vi "Ixon z-stack acquisition.vi"() -> ()   [LabVIEW 2015]
doc: "Acquires a z-stack of images using the Andor iXon camera and the piezo stage. The VI can be configured to sequentially acquire frames in multiple modes with different light sources and numbers of frames in each mode. Each mode is collected into a separate aquisition directory in Glimpse. Acquisition can be time-lapsed with a settable delay interval between cycles; the selected laser(s) are shuttered whilst not acquiring. The ixon setup acquisition.vi front panel is displayed so that the user can set the acquisition parameters before acquiring.\n\nThis is a Glimpse plug-in. To insure proper operation, you should have the source version of Glimpse running before loading this program. (The source version has an .llb extension, not a .exe one). Alternatively, the plug-in can be inserted into the executable version of Glimpse as a dynamically loaded VI."
uses:
  Glimpse core/Video acquisition state.ctl
  <vilib>/vision/Image Controls.llb/IMAQ Image.ctl
  Glimpse core/Seq file v 1/Offset table.ctl
  Glimpse core/Seq file v 1/file number.ctl
  Glimpse core/Seq file v 1/Offset.ctl
  Glimpse core/GLIMPSE Globals.vi
  ixon1024/camera defaults globals.vi
  Camera/camera globals.vi
  Stage/Move stage command.ctl
  ixon1024/ixon readout settings.ctl
  ixon1024/andor acquisition mode.ctl
  ixon1024/HAL camera parameters important.ctt
  new-h-nu-ixon/Laser type.ctt
  new-h-nu-ixon/Emission filters.ctl
panel:
  in  "Delay after\nfilter change\n(ms)":u32
  in  "Max. number of acquisition files":i8(slide)=10 scale=0.0..50.0
  in  "Camera Parameters":T1={"Exposure Time (sec)"=0.1, "EM CCD Gain"=230, "Readout Settings"={"Acquisition Mode"=enum."Frame Transfer Run till Abort", "Pixel Rate"=enum."EM CCD 5 Mhz 14 bits", "High Capacity?"=FALSE, "V Shift Speed (us/row)"=enum."6.5", "V Shift Amplitude"=enum."+1", "Preamp Gain"=enum."2.4", "Trigger Mode"=0, "Baseline offset"=0, "Baseline clamp"=FALSE}, "Image Size"={"H Bin"=1, "V Bin"=1, "Left"=1, "Top"=1, "Right"=1024, "Bottom"=730}} {"Readout Settings"."Baseline offset" min=-1000 max=1000 step=100; "Readout Settings"."Trigger Mode" items=["Internal", "External"]; "EM CCD Gain" scale=1.0..300.0; "Exposure Time (sec)" scale=0.001..10.0 scale format="%#_1g"}
  in  "stage settle time (ms)":u32=300
  in  "stack half-width (steps)":u32=8
  in  "focus step (um)":ext=0.150000000000000000005
  in  "Cycle Interval (s)":dbl format="%_3f"
  in  "Acquisition Protocol":T6(array[cluster])
  # "Z-stack parameters"
  # "Camera: Andor iXon"
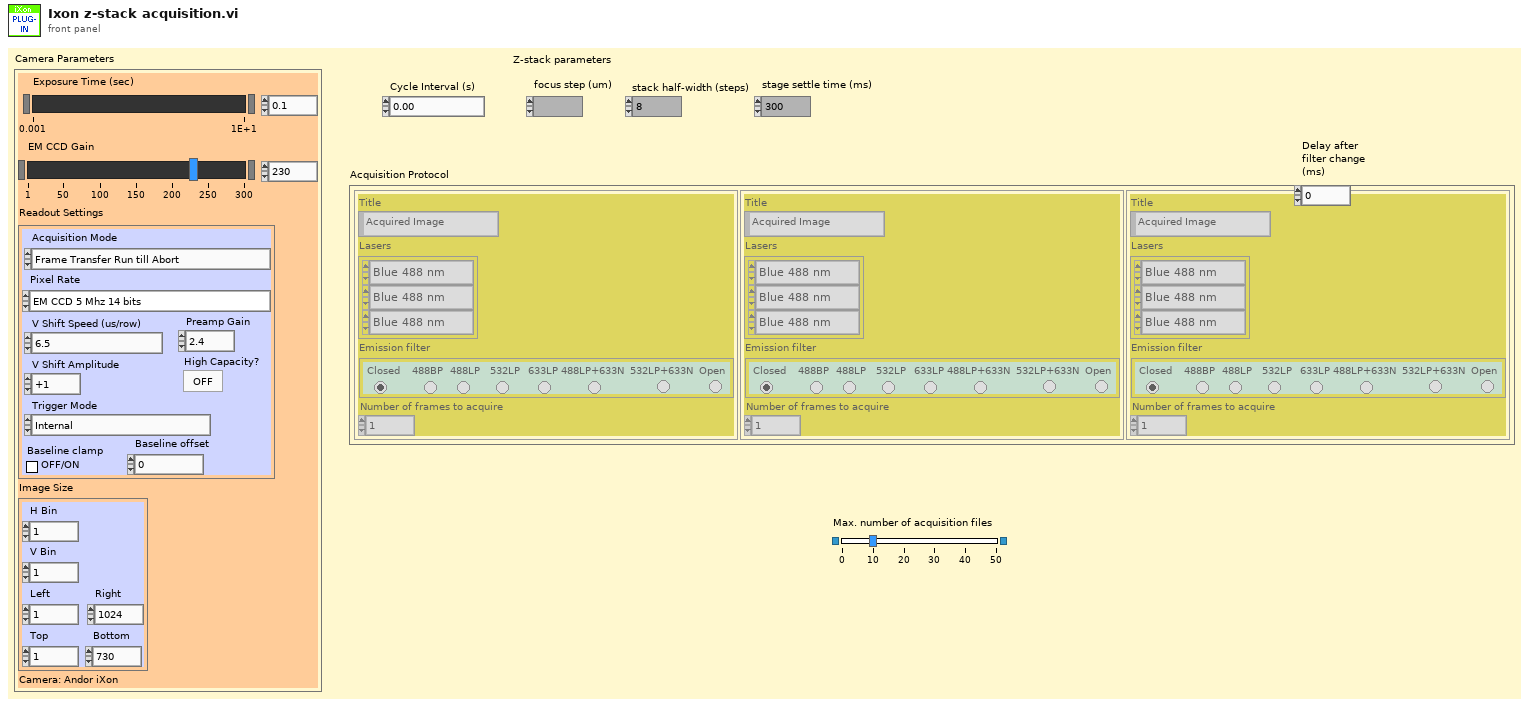
[diagram p1: front panel]
types:
  T1 = typedef "HAL camera parameters important.ctt" = cluster{"Exposure Time (sec)":sgl, "EM CCD Gain":u16, "Readout Settings":T2, "Image Size":cluster{"H Bin":i32, "V Bin":i32, "Left":i32, "Top":i32, "Right":i32, "Bottom":i32}}
  T2 = typedef "ixon readout settings.ctl" = cluster{"Acquisition Mode":T3, "Pixel Rate":enum16{"EM CCD 10 Mhz 14 bits", "EM CCD 5 Mhz 14 bits", "EM CCD 3 Mhz 14 bits", "EM CCD 1 Mhz 16 bits", "Standard CCD 3 Mhz 14 bits", "Standard CCD 1 Mhz 16 bits"}, "High Capacity?":bool, "V Shift Speed (us/row)":enum16{"0.9 (not reccommended)", "1.7  (not reccommended)", "3.3  (not reccommended)", "6.5", "12.9"}, "V Shift Amplitude":enum16{"normal", "+1", "+2", "+3", "+4"}, "Preamp Gain":enum16{"1.0", "2.4", "5.0"}, "Trigger Mode":u32, "Baseline offset":i16, "Baseline clamp":bool}
  T3 = typedef "andor acquisition mode.ctl" = enum16{"(do not use)", "Single Scan", "Accumulate", "Kinetics", "Fast Kinetics", "Kinetics Run till Abort", "Frame Transfer", "Frame Transfer Run till Abort", "(do not use) ", "Time Delayed Integration"}
  T4 = typedef "Laser type.ctt" = enum16{"Blue 488 nm", "Green 532 nm", "Red 633 nm", "IR 780"}
  T5 = typedef "Emission filters.ctl" = enum32{" Closed ", " 488BP ", "488LP", "  532LP ", "633LP", "488LP+633N", "532LP+633N", "Open"}
  T6 = cluster{"Title":string, "Lasers":T4[], "Emission filter":T5, "Number of frames to acquire":i32}[]
  T7 = typedef "image size.ctl" = cluster{"H Bin":i32, "V Bin":i32, "Left":i32, "Top":i32, "Right":i32, "Bottom":i32}
  T8 = typedef "Glimpse file parameters.ctt" = cluster{"Frame Size (bytes)":u32, "Max Frames":u32, "Max time (s)":u32, "Max Time (min)":u32, "Max Space Req'd. (Gb)":dbl, "Frames per acquisition file":u32}
  T9 = typedef "Move stage command.ctl" = cluster{"dx (um) (0 -> ignore)":ext, "dy (um) (0 -> ignore)":ext, "dz (um) (0 -> ignore)":ext, "Re-center x,y":bool, "Re-center z":bool, "x (um) (-1 -> ignore)":dbl, "y (um) (-1 -> ignore)":dbl, "z (um) (-1 -> ignore)":dbl}
  T10 = typedef "Video acquisition state.ctl" = cluster{"Pixel depth":enum32{"8 bits", "16 bits", "Float", "Complex", "RGB Chunky", "Compressed"}, "Width":dbl, "Height":dbl, "Buffer":T11, "Frames Acquired":u32, "Time of 1st frame":dbl, "TTB element zero":u32, "File Offsets Array":T12, "TTB Array":u32[], "Sum Image (for averaging)":T11, "Time at end of last acquisition (ms)":u32, "Filter array":u16[], "Flow rate array":dbl[], "Temperature array":dbl[], "Field array":u16[], "Lasers array":u16[][], "Stage xyz array":dbl[][]}
  T11 = typedef "IMAQ Image.ctl" = refnum<image>
  T12 = typedef "Offset table.ctl" = cluster{"offset":T13, "file number":T14}[]
  T13 = typedef "Offset.ctl" = i32
  T14 = typedef "file number.ctl" = u8
  T15 = typedef "Sequence files handle.ctt" = cluster{"Sequence files directory path":path, "Sequence files refnum array":refnum<file>[]}
  T16 = cluster{"dx (um)":ext, "dy (um)":ext, "dz (um)":ext}
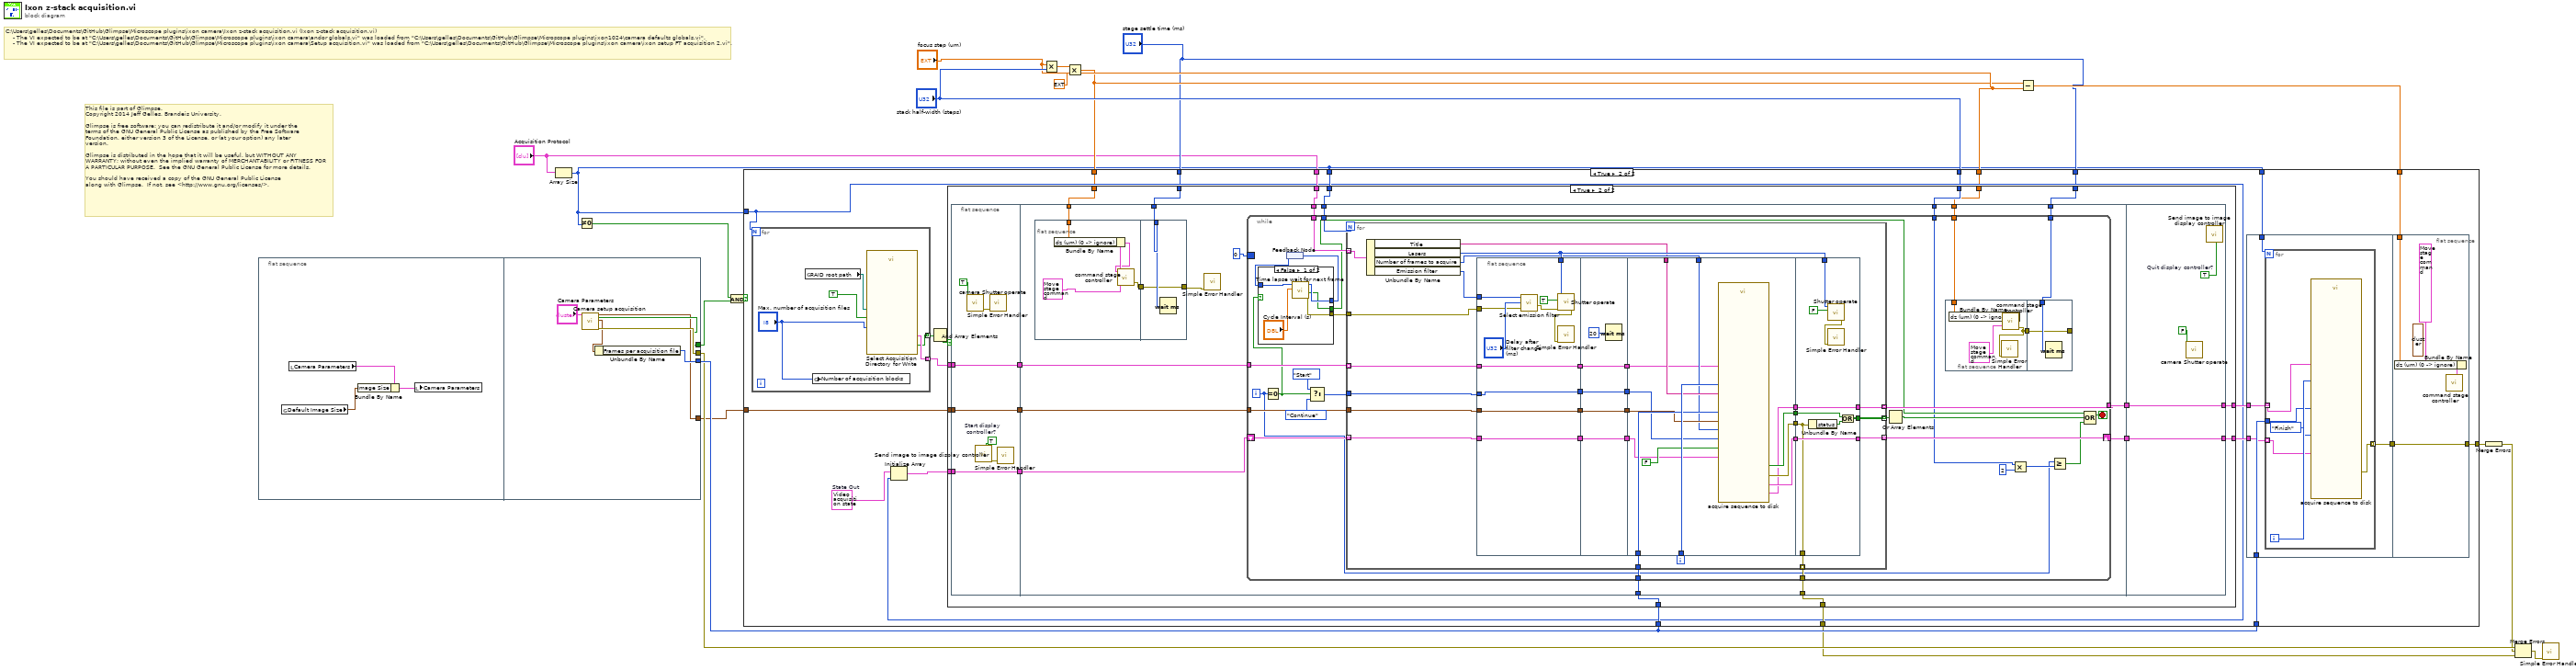
[diagram p0: block diagram]
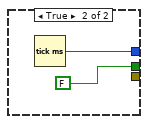
[diagram p4: hidden frame]
diagram:
  # "C:\\Users\\gelles\\Documents\\GitHub\\Glimpse\\Microscope plugins\\ixon camera\\Ixon z-stack acquisition.vi (Ixon z-stack acquisition.vi)\n    - The VI expected to be at \"C:\\Users\\gelles\\Documents\\GitHub\\Glimpse\\Microscope plugins\\ixon camera\\andor globals.vi\" was loaded from \"C:\\Users\\gelles\\Documents\\GitHub\\Glimpse\\Microscope plugins\\ixon1024\\camera defaults globals.vi\".\n    - The VI expected to be at \"C:\\Users\\gelles\\Documents\\GitHub\\Glimpse\\Microscope plugins\\ixon camera\\Setup acquisition.vi\" was loaded from \"C:\\Users\\gelles\\Documents\\GitHub\\Glimpse\\Microscope plugins\\ixon camera\\ixon setup FT acquisition 2.vi\"."
  # "This file is part of Glimpse. \nCopyright 2014 Jeff Gelles, Brandeis University.    \n\nGlimpse is free software: you can redistribute it and/or modify it under the \nterms of the GNU General Public License as published by the Free Software \nFoundation, either version 3 of the License, or (at your option) any later \nversion.\n\nGlimpse is distributed in the hope that it will be useful, but WITHOUT ANY \nWARRANTY; without even the implied warranty of MERCHANTABILITY or FITNESS FOR \nA PARTICULAR PURPOSE.  See the GNU General Public License for more details.\n\nYou should have received a copy of the GNU General Public License\nalong with Glimpse.  If not, see <http://www.gnu.org/licenses/>."
  n1 = flat-sequence {
    tunnel: [w24] -> w11
    tunnel: [w27] -> w10
    tunnel: [w26] -> w4
    tunnel: [w23] -> w1
    frame #0 {
      n2 = global read "camera defaults globals.vi" "Default Image Size"() -> (w22:T7)
      n3 = local read "Camera Parameters"() -> (w21:T1)
      n4 = Bundle By Name(cluster=w21, "Image Size"=w22) -> (w20:T1)
      n5 = local write "Camera Parameters"(w20) -> ()
    }
    frame #1 {
      n6 = call "Camera setup acquisition.vi"("Camera Parameters (important)"="Camera Parameters") -> ("Image Size Out"=w23:T7, "Continue with acq?"=w26:bool, "Glimpse file properties"=w25:T8, "Error Out (no error)"=w27:errorcluster)  [unwired: 6 in, 9 out]
      n7 = Unbundle By Name(w25) -> ("Frames per acquisition file"=w24:u32)
    }
  }
  n8 = Array Size(array="Acquisition Protocol") -> (size(s)=w3:i32)
  n9 = Not Equal To 0?(x=w3) -> (x != 0?=w2:bool)
  n10 = And(x=w2, y=w4) -> (x .and. y?=w5:bool)
  n11 = Multiply(x="focus step (um)", y="stack half-width (steps)") -> (x*y=w19:ext)
  n12 = Multiply(x=w19, y=ext -1.0) -> (x*y=w14:ext)
  n13 = Subtract(x=w14, y="focus step (um)") -> (x-y=w15:ext)
  n14 = case shown="True" w5 {
    tunnel: w11 -> [_ w50]
    tunnel: w11 -> [_ w49]
    tunnel: [_ w48] -> w8
    tunnel: [_ w47] -> w9
    tunnel: w3 -> [_ w37]
    tunnel: w3 -> [_ w43]
    tunnel: w3 -> [_ w40]
    tunnel: "Acquisition Protocol" -> [_ w38]
    tunnel: w1 -> [_ w36]
    tunnel: "stack half-width (steps)" -> [_ w35]
    tunnel: "stage settle time (ms)" -> [_ w34]
    tunnel: "focus step (um)" -> [_ w33]
    tunnel: w15 -> [_ w31]
    tunnel: w14 -> [_ w30]
    tunnel: "stage settle time (ms)" -> [_ w29]
    frame False {
    }
    frame True {
      w42 = T10 {"Pixel depth"=enum."8 bits", "Width"=0.0, "Height"=0.0, "Buffer"=refnum, "Frames Acquired"=0, "Time of 1st frame"=0.0, "TTB element zero"=0, "File Offsets Array"=[], "TTB Array"=[], "Sum Image (for averaging)"=refnum, "Time at end of last acquisition (ms)"=0, "Filter array"=[], "Flow rate array"=[], "Temperature array"=[], "Field array"=[], "Lasers array"=[], "Stage xyz array"=[]}  # State Out
      n15 = for {
        N: w37 -> [_]
        tunnel: [w231] -> w39 mode=indexing
        tunnel: [w230] -> w51 mode=indexing
        n16 = global read "GLIMPSE Globals.vi" "RAID root path"() -> (w233:path)
        n17 = global write "camera globals.vi" "Number of acquisition blocks"("Max. number of acquisition files") -> ()
        n18 = call "Select Acquisition Directory for Write.vi"("Autostart?"=TRUE, "Acquisition directory root path"=w233, "Number of acquisition files"="Max. number of acquisition files") -> ("Sequence files handle"=w231:T15, "OK?"=w230:bool)  [unwired: 11 in]
      }
      n19 = Initialize Array(w42, w37) -> (w41:T10[])
      n20 = And Array Elements(Boolean array=w51) -> (logical AND=w44:bool)
      n21 = case shown="True" w44 {
        tunnel: [w67 w87] -> w46
        tunnel: w39 -> [w67 w86]
        tunnel: w50 -> [_ w85]
        tunnel: [w68 w84] -> w45
        tunnel: [_ w83] -> w48
        tunnel: w43 -> [_ w82]
        tunnel: w41 -> [w68 w81]
        tunnel: w38 -> [_ w80]
        tunnel: w36 -> [_ w75]
        tunnel: w35 -> [_ w73]
        tunnel: w34 -> [_ w72]
        tunnel: w33 -> [_ w71]
        tunnel: w30 -> [_ w70]
        tunnel: w29 -> [_ w69]
        frame False {
        }
        frame True {
          n22 = flat-sequence {
            tunnel: w81 -> [w93]
            tunnel: w86 -> [w94]
            tunnel: [w94] -> w79
            tunnel: [w93] -> w78
            tunnel: w75 -> [w91]
            tunnel: [w91] -> w74
            tunnel: w85 -> [w109]
            tunnel: [w107] -> w83
            tunnel: w82 -> [w106]
            tunnel: w80 -> [w104]
            tunnel: w79 -> [w110]
            tunnel: w78 -> [w105]
            tunnel: [w111] -> w77
            tunnel: [w108] -> w76
            tunnel: w74 -> [w102]
            tunnel: w73 -> [w101]
            tunnel: w72 -> [w100]
            tunnel: w71 -> [w99]
            tunnel: w70 -> [w97]
            tunnel: w69 -> [w96]
            tunnel: [w227] -> w84
            tunnel: [w228] -> w87
            tunnel: w77 -> [w228]
            tunnel: w76 -> [w227]
            frame #0 {
              w90 = TRUE  # Start display  controller?
              n23 = call "camera Shutter operate.vi"("Open?"=TRUE) -> ("error out"=w88:errorcluster)  [unwired: 7 in]
              n24 = call "Send image to image display controller.vi"("Start display controller?"=w90) -> ("error out"=w89:errorcluster)  [unwired: 8 in, 1 out]
              n25 = call <vilib>:"Simple Error Handler.vi"("error in (no error)"=w88) -> ()  [unwired: 4 in, 5 out]
              n26 = call <vilib>:"Simple Error Handler.vi"("error in (no error)"=w89) -> ()  [unwired: 4 in, 5 out]
            }
            frame #1 {
              n27 = flat-sequence {
                tunnel: w97 -> [w112]
                tunnel: [w115] -> w98
                tunnel: w96 -> [w117]
                tunnel: [w116] -> w95
                tunnel: w98 -> [w116]
                frame #0 {
                  n28 = Bundle By Name(cluster=T9 {"dx (um) (0 -> ignore)"=0.0, "dy (um) (0 -> ignore)"=0.0, "dz (um) (0 -> ignore)"=0.0, "Re-center x,y"=FALSE, "Re-center z"=FALSE, "x (um) (-1 -> ignore)"=-1.0, "y (um) (-1 -> ignore)"=-1.0, "z (um) (-1 -> ignore)"=-1.0} ("command"), "dz (um) (0 -> ignore)"=w112) -> (w113:T9)
                  n29 = call "command stage controller.vi"("command"=w113) -> ("error out"=w115:errorcluster)  [unwired: 7 in]
                }
                frame #1 {
                  n30 = Wait (ms)(milliseconds to wait=w117) -> ()  [unwired: 1 out]
                }
              }
              n31 = call <vilib>:"Simple Error Handler.vi"("error in (no error)"=w95) -> ()  [unwired: 4 in, 5 out]
              n32 = while {
                tunnel: [w145] -> w111
                tunnel: w110 -> [w144]
                tunnel: w109 -> [w143]
                shift-right: [w141] -> w108
                shift-left: w105 -> [w142]
                tunnel: [w140] -> w107
                tunnel: w106 -> [w135]
                tunnel: w104 -> [w134]
                tunnel: w102 -> [w129]
                tunnel: w101 -> [w121]
                tunnel: w100 -> [w119]
                tunnel: w99 -> [w118]
                border: u32 0 -> [_]
                i -> [w126]
                stop <- w125 stop-if-true
                n33 = Equal To 0?(x=w126) -> (x = 0?=w133:bool)
                n34 = feedback #1() -> (w131:u32)
                n35 = case shown="False" w133 {
                  tunnel: [w156 w158] -> w132
                  tunnel: [w155 FALSE] -> w124
                  tunnel: w131 -> [w154 _]
                  tunnel: [w152 _] -> w130
                  frame False {
                    n36 = call "Time lapse wait for next frame.vi"("Frame Interval (s)"="Cycle Interval (s)", "Time of last frame in"=w154) -> ("error out"=w152:errorcluster, "Stopped?"=w155:bool, "Time of this frame out (ms)"=w156:u32)  [unwired: 4 in, 1 out]
                  }
                  frame True {
                    n37 = Tick Count (ms)() -> (millisecond timer value=w158:u32)
                  }
                }
                n38 = feedback-in #1(w132) -> ()
                n39 = Select(t=enum16{"Start", "Continue", "Finish"}."Start" ("Operation"), s=w133, f=enum16{"Start", "Continue", "Finish"}."Continue" ("Operation")) -> (s? t:f=w137:enum16{"Start", "Continue", "Finish"})
                n40 = for {
                  N: w135 -> [_]
                  tunnel: [w180] -> w145 mode=indexing
                  tunnel: w144 -> [w179] mode=indexing
                  tunnel: w143 -> [w178]
                  tunnel: w142 -> [w171] mode=indexing
                  tunnel: [w177] -> w141 mode=indexing
                  tunnel: [w176] -> w136 mode=indexing
                  tunnel: [w175] -> w140 mode=indexing
                  tunnel: w137 -> [w174]
                  tunnel: w134 -> [w168] mode=indexing
                  tunnel: w130 -> [w163]
                  tunnel: w129 -> [w162]
                  i -> [w165]
                  n41 = Unbundle By Name(w168) -> ("Title"=w164:string, "Lasers"=w167:T4[], "Number of frames to acquire"=w166:i32, "Emission filter"=w159:T5)
                  n42 = flat-sequence {
                    tunnel: w179 -> [w197]
                    tunnel: [w197] -> w186
                    tunnel: w167 -> [w194]
                    tunnel: w174 -> [w193]
                    tunnel: [w193] -> w172
                    tunnel: w171 -> [w192]
                    tunnel: [w192] -> w169
                    tunnel: w163 -> [w189]
                    tunnel: w162 -> [w191]
                    tunnel: [w191] -> w161
                    tunnel: w159 -> [w187]
                    tunnel: w186 -> [w202]
                    tunnel: [w202] -> w185
                    tunnel: [w200] -> w173
                    tunnel: w172 -> [w200]
                    tunnel: [w199] -> w170
                    tunnel: w169 -> [w199]
                    tunnel: w161 -> [w198]
                    tunnel: [w198] -> w160
                    tunnel: w185 -> [w204]
                    tunnel: [w205] -> w184
                    tunnel: [w203] -> w183
                    tunnel: [w206] -> w182
                    tunnel: w178 -> [w213]
                    tunnel: [w207] -> w181
                    tunnel: w173 -> [w210]
                    tunnel: w170 -> [w208]
                    tunnel: w166 -> [w211]
                    tunnel: w165 -> [w215]
                    tunnel: w164 -> [w214]
                    tunnel: w160 -> [w212]
                    tunnel: [w223] -> w180
                    tunnel: [w224] -> w177
                    tunnel: w184 -> [w224]
                    tunnel: w183 -> [w223]
                    tunnel: w182 -> [w217]
                    tunnel: w181 -> [w219]
                    tunnel: [w218] -> w176
                    tunnel: [w217] -> w175
                    tunnel: w167 -> [w216]
                    frame #0 {
                      n43 = call "Select emission filter.vi"("Emission filter"=w187, "Time to wait\nafter filter change\n(ms)"="Delay after\nfilter change\n(ms)", "error in"=w189) -> ("error out"=w188:errorcluster)  [unwired: 3 out]
                      n44 = call "Shutter operate.vi"("Shutters"=w194, 2:TRUE ("Data to Write"), "error in"=w188) -> ("error out"=w195:errorcluster)  [unwired: 5 in]
                      n45 = call <vilib>:"Simple Error Handler.vi"("error in (no error)"=w195) -> ()  [unwired: 4 in, 5 out]
                    }
                    frame #1 {
                      n46 = Wait (ms)(milliseconds to wait=u32 20) -> ()  [unwired: 1 out]
                    }
                    frame #2 {
                      n47 = call "acquire sequence to disk.vi"("Image Size"=w212, "State In"=w208, "Frames per acquisition file"=w213, "Sequence files handle"=w204, "Pressing stop automatically runs finish?"=FALSE, "Display Window Title"=w214, "Operation"=w210, "Display Window Number"=w215, "Number of frames to acquire"=w211) -> ("Done?"=w207:bool, "State Out"=w205:T10, "Sequence files handle out"=w203:T15, "error out"=w206:errorcluster)  [unwired: 7 in]
                    }
                    frame #3 {
                      n48 = Unbundle By Name(w217) -> ("status"=w220:bool)
                      n49 = call "Shutter operate.vi"("Shutters"=w216, 2:FALSE ("Data to Write")) -> ("error out"=w222:errorcluster)  [unwired: 6 in]
                      n50 = call <vilib>:"Simple Error Handler.vi"("error in (no error)"=w222) -> ()  [unwired: 4 in, 5 out]
                      n51 = Or(x=w219, y=w220) -> (x .or. y?=w218:bool)
                    }
                  }
                }
                n52 = Or Array Elements(Boolean array=w136) -> (logical OR=w123:bool)
                n53 = flat-sequence {
                  tunnel: w118 -> [w149]
                  tunnel: [w147] -> w120
                  tunnel: w119 -> [w151]
                  tunnel: [w150] -> _
                  tunnel: w120 -> [w150]
                  frame #0 {
                    n54 = Bundle By Name(cluster=T9 {"dx (um) (0 -> ignore)"=0.0, "dy (um) (0 -> ignore)"=0.0, "dz (um) (0 -> ignore)"=0.0, "Re-center x,y"=FALSE, "Re-center z"=FALSE, "x (um) (-1 -> ignore)"=-1.0, "y (um) (-1 -> ignore)"=-1.0, "z (um) (-1 -> ignore)"=-1.0} ("command"), "dz (um) (0 -> ignore)"=w149) -> (w148:T9)
                    n55 = call "command stage controller.vi"("command"=w148) -> ("error out"=w147:errorcluster)  [unwired: 7 in]
                    n56 = call <vilib>:"Simple Error Handler.vi"("error in (no error)"=w147) -> ()  [unwired: 4 in, 5 out]
                  }
                  frame #1 {
                    n57 = Wait (ms)(milliseconds to wait=w151) -> ()  [unwired: 1 out]
                  }
                }
                n58 = Multiply(x=w121, y=u32 2) -> (x*y=w127:u32)
                n59 = Greater Or Equal?(x=w126, y=w127) -> (x >= y?=w122:bool)
                n60 = Compound Arithmetic op=OR(w124, w123, w122) -> (w125:bool)
              }
            }
            frame #2 {
              w226 = TRUE  # Quit display controller?
              n61 = call "camera Shutter operate.vi"("Open?"=FALSE) -> ()  [unwired: 7 in, 1 out]
              n62 = call "Send image to image display controller.vi"("Quit display controller?"=w226) -> ()  [unwired: 8 in, 2 out]
            }
          }
        }
      }
      n63 = flat-sequence {
        tunnel: w49 -> [w56]
        tunnel: w46 -> [w54]
        tunnel: w45 -> [w53]
        tunnel: w40 -> [w52]
        tunnel: [w55] -> w32
        tunnel: [w66] -> w47
        tunnel: w32 -> [w66]
        tunnel: w31 -> [w64]
        frame #0 {
          n64 = for {
            N: w52 -> [_]
            tunnel: w56 -> [w60]
            tunnel: [w57] -> w55 mode=indexing
            tunnel: w54 -> [w62] mode=indexing
            tunnel: w53 -> [w58] mode=indexing
            i -> [w61]
            n65 = call "acquire sequence to disk.vi"("State In"=w58, "Frames per acquisition file"=w60, "Sequence files handle"=w62, "Operation"=enum16{"Start", "Continue", "Finish"}."Finish", "Display Window Number"=w61) -> ("error out"=w57:errorcluster)  [unwired: 11 in, 3 out]
          }
        }
        frame #1 {
          (unwired) T16 {"dx (um)"=0.0, "dy (um)"=0.0, "dz (um)"=0.0} ("command")
          n66 = Bundle By Name(cluster=T9 {"dx (um) (0 -> ignore)"=0.0, "dy (um) (0 -> ignore)"=0.0, "dz (um) (0 -> ignore)"=0.0, "Re-center x,y"=FALSE, "Re-center z"=FALSE, "x (um) (-1 -> ignore)"=-1.0, "y (um) (-1 -> ignore)"=-1.0, "z (um) (-1 -> ignore)"=-1.0} ("command"), "dz (um) (0 -> ignore)"=w64) -> (w65:T9)
          n67 = call "command stage controller.vi"("command"=w65) -> ()  [unwired: 7 in, 1 out]
        }
      }
    }
  }
  n68 = Merge Errors(w9) -> (w7:errorcluster)
  n69 = Merge Errors(w10, w7, w8) -> (w12:errorcluster)
  n70 = call <vilib>:"Simple Error Handler.vi"("error in (no error)"=w12) -> ()  [unwired: 4 in, 5 out]
